vi "plot_dataSubset_XY.vi"(1 "X-data":sgl[](array[numeric]), 3 "zoom range low":ext format="%.2f", 4 "zoom range high":sgl format="%.2f", 5 "error in (no error)":errorcluster) -> (14 "idx start":i32, 15 "length":i32, 17 "X min actual":sgl format="%.2f", 18 "X max actual":sgl format="%.2f", 19 "error out":errorcluster)   [LabVIEW 2010, in "OSA.lvclass"]
doc: "SubVI to a <B>Thorlabs_OSA_64</B> object.\n\n[GOOP 1.0]"
uses:
  OSA.lvclass
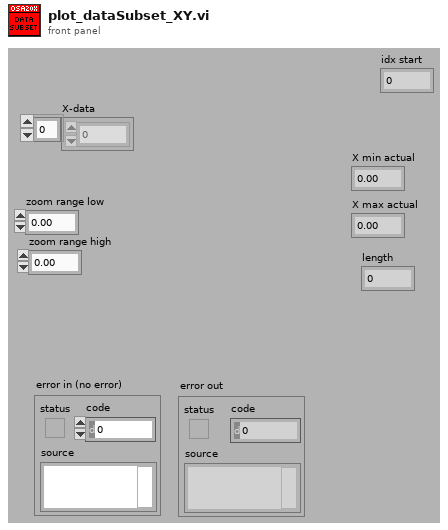
[diagram p1: front panel]
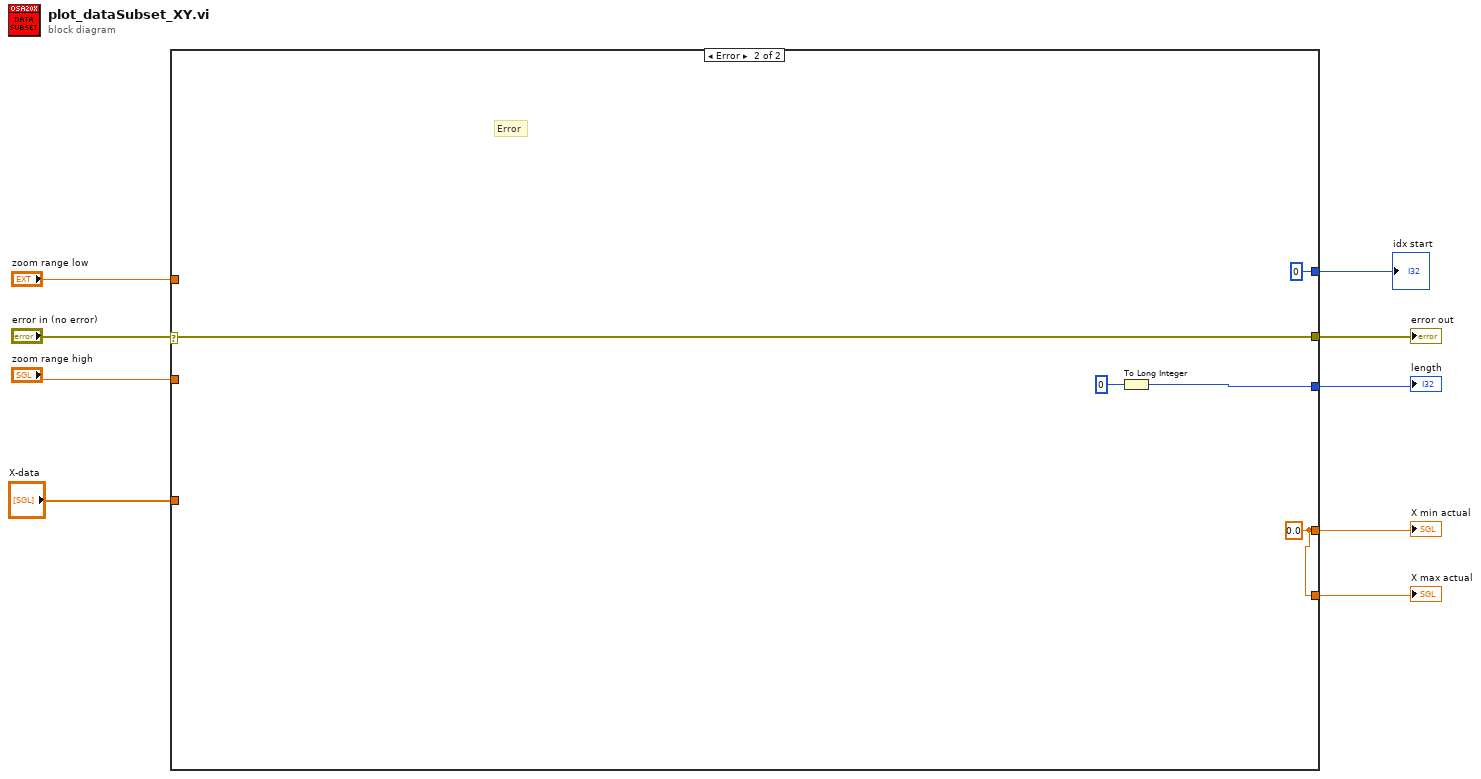
[diagram p0: block diagram]
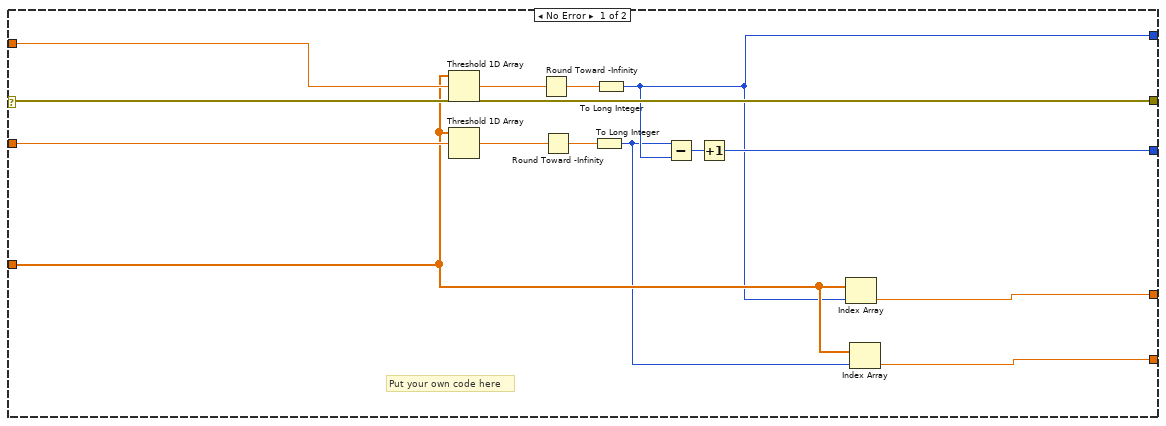
[diagram p2: hidden frame]
diagram:
  n1 = case shown="Error" "error in (no error)" {
    selector: "error in (no error)" -> [w23 w28]
    tunnel: [w23 w28] -> w9
    tunnel: "X-data" -> [w14 _]
    tunnel: "zoom range low" -> [w22 _]
    tunnel: "zoom range high" -> [w21 _]
    tunnel: [w17 w24] -> w4
    tunnel: [w15 w26] -> w3
    tunnel: [w18 w24] -> w2
    tunnel: [w11 0] -> w1
    frame No Error {
      # "Put your own code here"
      n2 = Threshold 1D Array(2:w22, 3:w14) -> (0:w12:sgl)  [unwired: 1 in]
      n3 = Threshold 1D Array(2:w21, 3:w14) -> (0:w13:sgl)  [unwired: 1 in]
      n4 = Round Toward -Infinity(1:w12) -> (0:w20:sgl)
      n5 = Round Toward -Infinity(1:w13) -> (0:w19:sgl)
      n6 = To Long Integer(number=w19) -> (32bit integer=w10:i32)
      n7 = To Long Integer(number=w20) -> (32bit integer=w11:i32)
      n8 = Subtract(x=w10, y=w11) -> (x-y=w16:i32)
      n9 = Increment(x=w16) -> (x+1=w15:i32)
      n10 = Index Array(array=w14, index=w11) -> (element=w18:sgl)
      n11 = Index Array(array=w14, index=w10) -> (element=w17:sgl)
    }
    frame Error {
      w24 = sgl 0.0 ("Numeric")
      # "Error"
      n12 = To Long Integer(number=0) -> (32bit integer=w26:i32)
    }
  }
  "error out" <- w9
  "X min actual" <- w2
  "X max actual" <- w4
  "length" <- w3
  "idx start" <- w1
